vi "ins_subq.vi"(0 "data":T2, 1 "table_name":string, 2 "columns":string[](array[string]), 3 "error out":errorcluster, 4 "conn ref out":T1) -> (5 "connection reference out":T1, 6 "error out 2":errorcluster)   [LabVIEW 2010]
uses:
  <vilib>/addons/database/Connection.llb/Conn ObjectReference.ctl
  <vilib>/addons/database/NI_Database_API.lvlib
panel:
  in  "Case Constant\n(See Context Help) 2":bool=TRUE
  in  "Case Constant\n(See Context Help)":bool
  out "resulting string":string
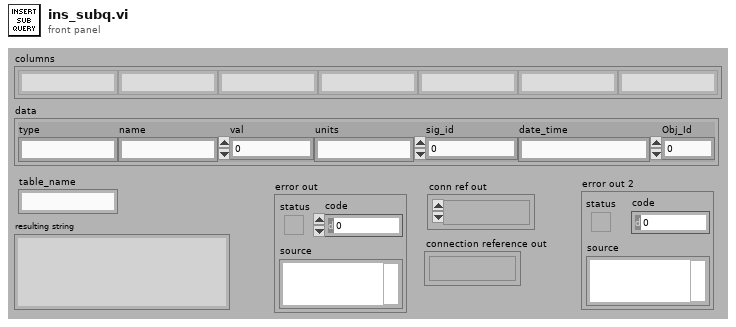
[diagram p1: front panel]
types:
  T1 = typedef "NI_Database_API.lvlib/Conn ObjectReference.ctl" = refnum<k1>
  T2 = cluster{"type":string, "name":string, "val":dbl, "units":string, "sig_id":i32, "date_time":string, "Obj_Id":i32}
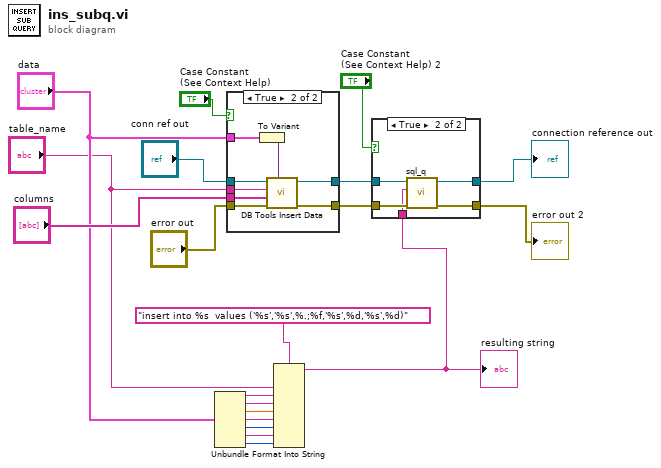
[diagram p0: block diagram]
diagram:
  n1 = Unbundle("data") -> ("type"=w14:string, "name"=w13:string, "val"=w12:dbl, "units"=w11:string, "sig_id"=w10:i32, "date_time"=w9:string, "Obj_Id"=w8:i32)
  n2 = case shown="True" "Case Constant\n(See Context Help)" {
    tunnel: "error out" -> [w21 w30]
    tunnel: "conn ref out" -> [w22 w29]
    tunnel: "columns" -> [_ w27]
    tunnel: [w22 w26] -> w5
    tunnel: [w21 w25] -> w3
    tunnel: "data" -> [_ w24]
    tunnel: "table_name" -> [_ w23]
    frame False {
    }
    frame True {
      n3 = To Variant(anything=w24) -> (Variant=w28:variant)
      n4 = call <vilib>:"DB Tools Insert Data.vi"("data"=w28, "error in (no error)"=w30, "columns"=w27, "table"=w23, "connection reference"=w29) -> ("error out"=w25:errorcluster, "connection reference out"=w26:T1)  [unwired: 5 in]
    }
  }
  n5 = Format Into String(format string="insert into %s  values ('%s','%s',%.;%f,'%s',%d,'%s',%d)", "table_name", w14, w13, w12, w11, w10, w9, w8) -> (resulting string=w1:string)  [unwired: 2 in, 1 out]
  "resulting string" <- w1
  n6 = case shown="True" "Case Constant\n(See Context Help) 2" {
    tunnel: w3 -> [w31 w37]
    tunnel: [w31 w36] -> w2
    tunnel: [w32 w35] -> w4
    tunnel: w5 -> [w32 w34]
    tunnel: w1 -> [_ w33]
    frame False {
    }
    frame True {
      n7 = call "sql_q.vi"("error in"=w37, "SQL query"=w33, "connect ref"=w34) -> ("error out"=w36:errorcluster, "conn ref out"=w35:T1)  [unwired: 1 in, 2 out]
    }
  }
  "connection reference out" <- w4
  "error out 2" <- w2
